vi "splitt formulas.vi"(1 "formula":string="(v1*3+4,,5)") -> (0 "Array":string[](array[string])=["1*3+4", "", "5"])   [LabVIEW 2011]
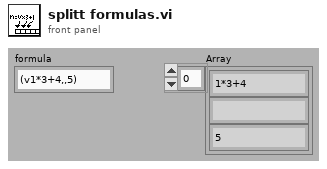
[diagram p1: front panel]
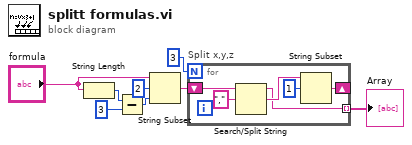
[diagram p0: block diagram]
diagram:
  n1 = String Length(string="formula") -> (length=w2:i32)
  n2 = Subtract(x=w2, y=3) -> (x-y=w4:i32)
  n3 = String Subset(string="formula", offset (0)=2, length (rest)=w4) -> (substring=w5:string)
  n4 = for "Split x,y,z" {
    N: 3 -> [_]
    shift-right: [w11] -> _
    shift-left: w5 -> [w14]
    tunnel: [w9] -> w7 mode=indexing
    n5 = Search/Split String(string=w14, search string/char (-)=",") -> (substring before match=w9:string, match + rest of string=w12:string)  [unwired: 1 in, 1 out]
    n6 = String Subset(string=w12, offset (0)=1) -> (substring=w11:string)  [unwired: 1 in]
  }
  "Array" <- w7
